vi "write general keywords.vi"(8 "error in (no error)":errorcluster, 11 "Save Image in":refnum<class "Save Image.lvclass">) -> (0 "error out":errorcluster, 3 "Save Image out":refnum<class "Save Image.lvclass">)   [LabVIEW 2018, in "Save Image.lvclass"]
uses:
  Save Image.lvclass
  Save Image.lvclass/Save Image.ctl
  Channel/Channel.lvclass/Channel.ctl
  Simulated_CCD_Camera/Simulated Camera.lvclass
  Channel/Channel.lvclass
panel:
  in  "Channel information":T1
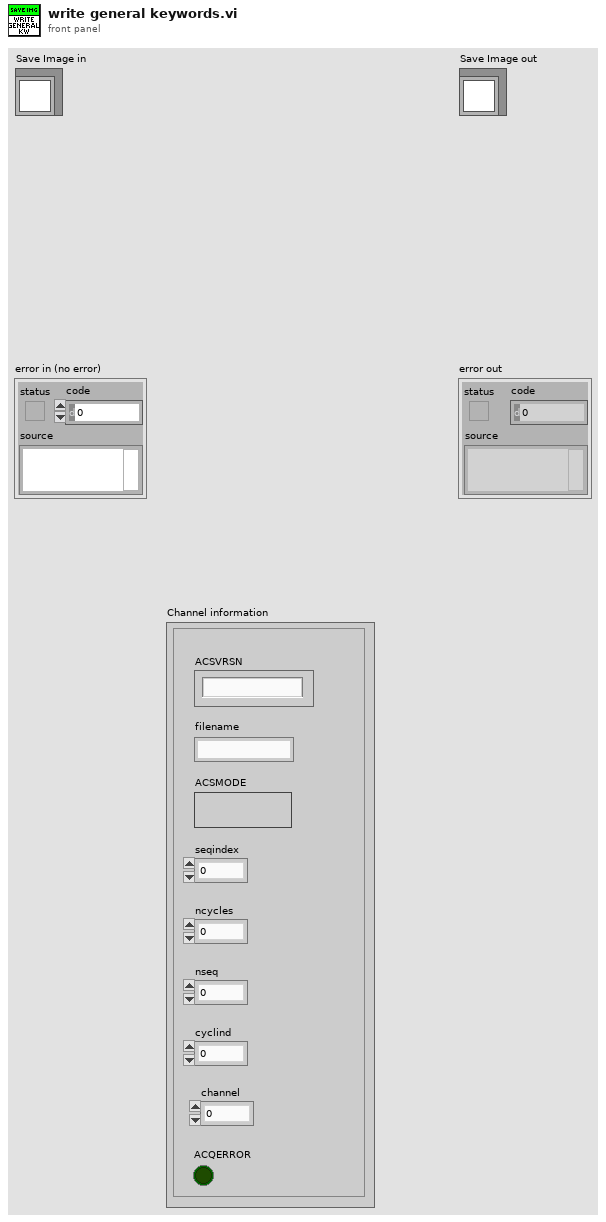
[diagram p1: front panel]
types:
  T1 = cluster{"ACSVRSN":string, "ACSMODE":bool, "filename":string, "seqindex":u16, "ncycles":u16, "nseq":u16, "cyclind":u16, "channel":u16, "ACQERROR":bool}
  T2 = cluster{"Image path":path, "Channel":u8, "S4ACS mode":u16, "Log file path":path, "log level":u16}
  T3 = cluster{"suffix":string, "#CYCLES":u32, "#SEQS":u32, "WAVEPLATE_POS":u16, "Waveplate positions":u8[]}
  T4 = cluster{"CYCLES_DONE":u16, "LAST_IMAGE_NAME":string, "USED_DISK_SPACE":u16, "FRAMES_DONE":u16, "CCD_STATUS":string, "CURRENT_TEMPERATURE":i16, "TEMPERATURE_STATUS":string, "FRAME_EXPOSURE_TIME":sgl, "ERROR":bool, "SERIAL_NUMBER":u16, "ACQUIRING":bool, "IMAGE_INDEX":u32, "SEQS_DONE":u16}
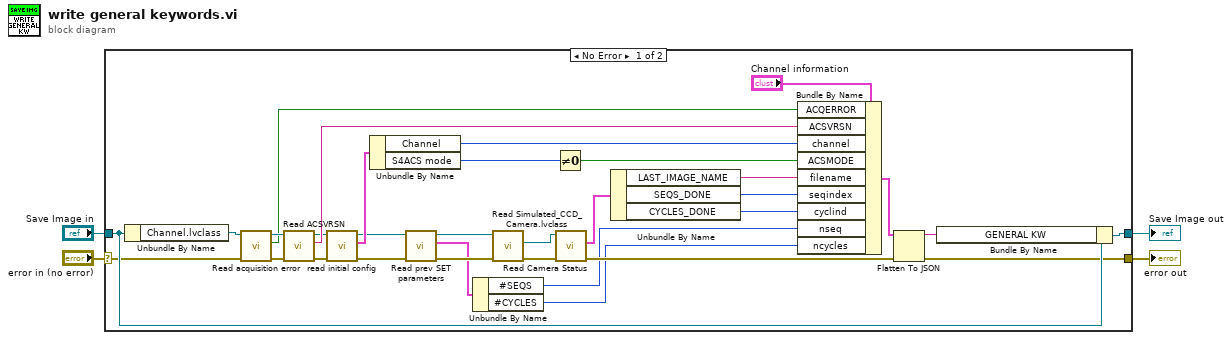
[diagram p0: block diagram]
diagram:
  n1 = case shown="No Error" "error in (no error)" {
    selector: "error in (no error)" -> [w13 w38]
    tunnel: [w25 w38] -> w3
    tunnel: [w22 w37] -> w1
    tunnel: "Save Image in" -> [w26 w37]
    frame No Error {
      n2 = Unbundle By Name(w26) -> ("Channel.lvclass"=w16:refnum<class "Channel.lvclass">)
      n3 = call-dynamic "Read acquisition error.vi"("error in (no error)"=w13, "Channel in"=w16) -> ("error out"=w14:errorcluster, "acquisition error"=w12:bool, "Channel out"=w15:refnum<class "Channel.lvclass">)  [unwired: 7 in]
      n4 = call "Read ACSVRSN.vi"("error in (no error)"=w14, "Channel in"=w15) -> ("error out"=w18:errorcluster, "ACSVRSN"=w35:string, "Channel out"=w19:refnum<class "Channel.lvclass">)  [unwired: 7 in]
      n5 = call-dynamic "read initial config.vi"("error in (no error)"=w18, "Channel in"=w19) -> ("error out"=w8:errorcluster, "Configuration to initialize ACS"=w36:T2, "Channel out"=w11:refnum<class "Channel.lvclass">)  [unwired: 7 in]
      n6 = Unbundle By Name(w36) -> ("Channel"=w17:u8, "S4ACS mode"=w20:u16)
      n7 = call-dynamic "Read prev SET parameters.vi"("error in (no error)"=w8, "Channel in"=w11) -> ("error out"=w9:errorcluster, "prev SET parameters"=w7:T3, "Channel out"=w10:refnum<class "Channel.lvclass">)  [unwired: 7 in]
      n8 = Unbundle By Name(w7) -> ("#SEQS"=w6:u32, "#CYCLES"=w5:u32)
      n9 = call "Read Simulated_CCD_Camera.lvclass.vi"("error in (no error)"=w9, "Channel in"=w10) -> ("error out"=w33:errorcluster, "Simulated_CCD_Camera.lvclass"=w34:refnum<class "Simulated Camera.lvclass">)  [unwired: 7 in, 1 out]
      n10 = Not Equal To 0?(x=w20) -> (x != 0?=w21:bool)
      n11 = call "Read Camera Status.vi"("error in (no error)"=w33, "CCDCamera in"=w34) -> ("error out"=w32:errorcluster, "Camera Status"=w31:T4)  [unwired: 7 in, 1 out]
      n12 = Unbundle By Name(w31) -> ("LAST_IMAGE_NAME"=w30:string, "SEQS_DONE"=w29:u16, "CYCLES_DONE"=w28:u16)
      n13 = Bundle By Name(cluster="Channel information", "ACQERROR"=w12, "ACSVRSN"=w35, "channel"=w17, "ACSMODE"=w21, "filename"=w30, "seqindex"=w29, "cyclind"=w28, "nseq"=w6, "ncycles"=w5) -> (w23:T1)
      n14 = Flatten To JSON(anything=w23, error in (no error)=w32) -> (JSON string=w24:string, 11:w25:errorcluster)  [unwired: 1 in]
      n15 = Bundle By Name(cluster=w26, "GENERAL KW"=w24) -> (w22:refnum<class "Save Image.lvclass">)
    }
    frame Error {
    }
  }
  "error out" <- w3
  "Save Image out" <- w1
